vi "Actor Core.vi"(8 "Error In":errorcluster, 11 "CS++RTRootActor in":refnum<class "CS++RTRootActor.lvclass">) -> (0 "Error Out":errorcluster, 3 "Actor out":refnum<class "Actor.lvclass">)   [LabVIEW 2014, in "CS++RTRoot.lvlib" / "CS++RTRootActor.lvclass"]
doc: "(<B>Filename</B>: Actor Framework.lvlib:Actor.lvclass:Actor Core.vi)\n\nReceives messages to the actor, reacts to them, and initiates any error handling that may shut the actor down.\n\nDescendant classes may override this VI to append parallel tasks for the actor to complete while it handles messages. Overrides use the Call Parent Method node."
uses:
  CS++RTRootActor.lvclass
  <vilib>/ActorFramework/Actor/Actor.lvclass
  CS++RTWatchdog/CS++RTWatchdogActor.lvclass
  CS++RTSystemHealth/CS++RTSystemHealthActor.lvclass
  CS++RTRootActor.lvclass/CS++RTRootActor.ctl
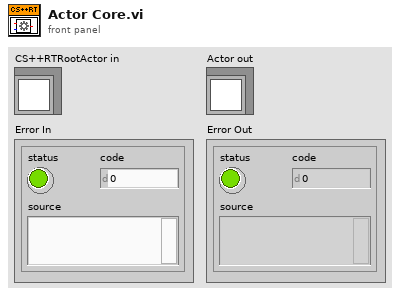
[diagram p1: front panel]
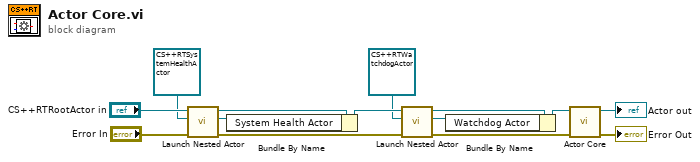
[diagram p0: block diagram]
diagram:
  n1 = call <vilib>:"Launch Nested Actor.vi"("error in (no error)"="Error In", "Nested Actor"=refnum<class "CS++RTSystemHealthActor.lvclass"> refnum ("CS++RTSystemHealth.lvlib:CS++RTSystemHealthActor.lvclass"), "Caller Actor in"="CS++RTRootActor in") -> ("error out"=w6:errorcluster, "Nested Actor's Enqueuer"=w12:refnum<class "Message Enqueuer.lvclass">, "Caller Actor out"=w10:refnum<class "CS++RTRootActor.lvclass">)  [unwired: 6 in]
  n2 = Bundle By Name(cluster=w10, "System Health Actor"=w12) -> (w5:refnum<class "CS++RTRootActor.lvclass">)
  n3 = call <vilib>:"Launch Nested Actor.vi"("error in (no error)"=w6, "Nested Actor"=refnum<class "CS++RTWatchdogActor.lvclass"> refnum ("CS++RTWatchdog.lvlib:CS++RTWatchdogActor.lvclass"), "Caller Actor in"=w5) -> ("error out"=w3:errorcluster, "Nested Actor's Enqueuer"=w7:refnum<class "Message Enqueuer.lvclass">, "Caller Actor out"=w8:refnum<class "CS++RTRootActor.lvclass">)  [unwired: 6 in]
  n4 = Bundle By Name(cluster=w8, "Watchdog Actor"=w7) -> (w2:refnum<class "CS++RTRootActor.lvclass">)
  n5 = call-parent "Actor Core.vi"("error in"=w3, "Actor in"=w2) -> ("error out"=→"Error Out":errorcluster, "Actor out"=→"Actor out":refnum<class "Actor.lvclass">)  [unwired: 8 in]
